vi "Keithley2450DrainS.vi"() -> ()   [LabVIEW 2025]
doc: "Author: Scott Hannahs <sth@magnet.fsu.edu>\n\nThis software is licensed for use under the “MIT License\"\nCopyright (c) 2025 Scott Hannahs, sth@sth@magnet.sthnet.net\n\nPermission is hereby granted, free of charge, to any person obtaining a copy of this software and associated documentation files (the \"Software\"), to deal in the Software without restriction, including without limitation the rights to use, copy, modify, merge, publish, distribute, sublicense, and/or sell copies of the Software, and to permit persons to whom the Software is furnished to do so, subject to the following conditions: The above copyright notice and this permission notice shall be included in all copies or substantial portions of the Software.\n\nTHE SOFTWARE IS PROVIDED \"AS IS\", WITHOUT WARRANTY OF ANY KIND, EXPRESS OR IMPLIED, INCLUDING BUT NOT LIMITED TO THE WARRANTIES OF MERCHANTABILITY, FITNESS FOR A PARTICULAR PURPOSE AND NONINFRINGEMENT. IN NO EVENT SHALL THE AUTHORS OR COPYRIGHT HOLDERS BE LIABLE FOR ANY CLAIM, DAMAGES OR OTHER LIABILITY, WHETHER IN AN ACTION OF CONTRACT, TORT OR OTHERWISE, ARISING FROM, OUT OF OR IN CONNECTION WITH THE SOFTWARE OR THE USE OR OTHER DEALINGS IN THE SOFTWARE."
panel:
  out "Sweep\nTime  (sec)":u32 format="%.1f"
  in  "Button:SetupBySoft":bool
  in  "Autozero:":bool
  out "Was paused":bool=TRUE
  in  "VISA resource name":refnum<visa-resource-name>="GPIB0::7::INSTR"
  in  "INFINITE RUN":bool
  in  "MODE:":enum32{"SAW /|/|/|", "TRINGLE /\\/\\/\\"}(radio)=enum."TRINGLE /\\/\\/\\"
  in  "Step |Volt| (abs.)":dbl=0.05 min=1e-06 max=0.1 format="%^.3e"
  in  "Delay (s)":dbl=1.0 min=0.1 max=100.0 format="%.3f"
  in  "Stop Volt":dbl=1.0 min=-10.0 max=10.0 format="%^.3e"
  in  "Start Sweep":bool
  out "Last index":i32
  in  "Compliance Current":dbl=0.1 format="%.3e"
  in  "Start Volt":dbl min=-10.0 max=10.0 format="%^.3e"
  in  "Setup":bool
  in  "Pause/Resume sweep":bool
  out "StartStorage":dbl min=-10.0 max=10.0 format="%^.3e"
  out "StopStorage":dbl=1.0 min=-10.0 max=10.0 format="%^.3e"
  in  "Button:Continue":bool
  in  "Button:SweepBySoft":bool
  out "Volt by Computer":dbl min=-10.0 max=10.0 format="%^.3e"
  in  "stop sweep":bool
  in  "Output Zero":bool
  # "Select name then start VI"
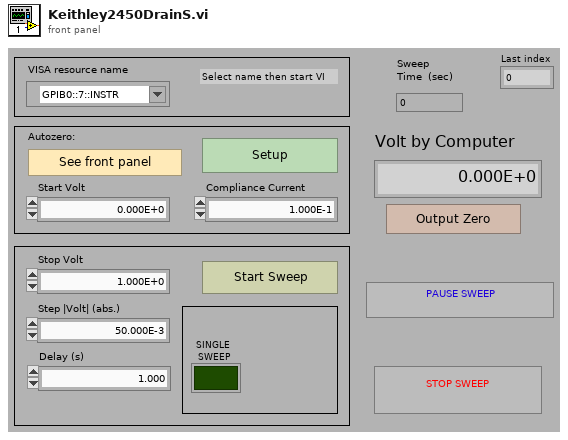
[diagram p1: front panel]
types:
  T1 = enum8{"Enabled", "Disabled", "Disabled and Grayed Out"}
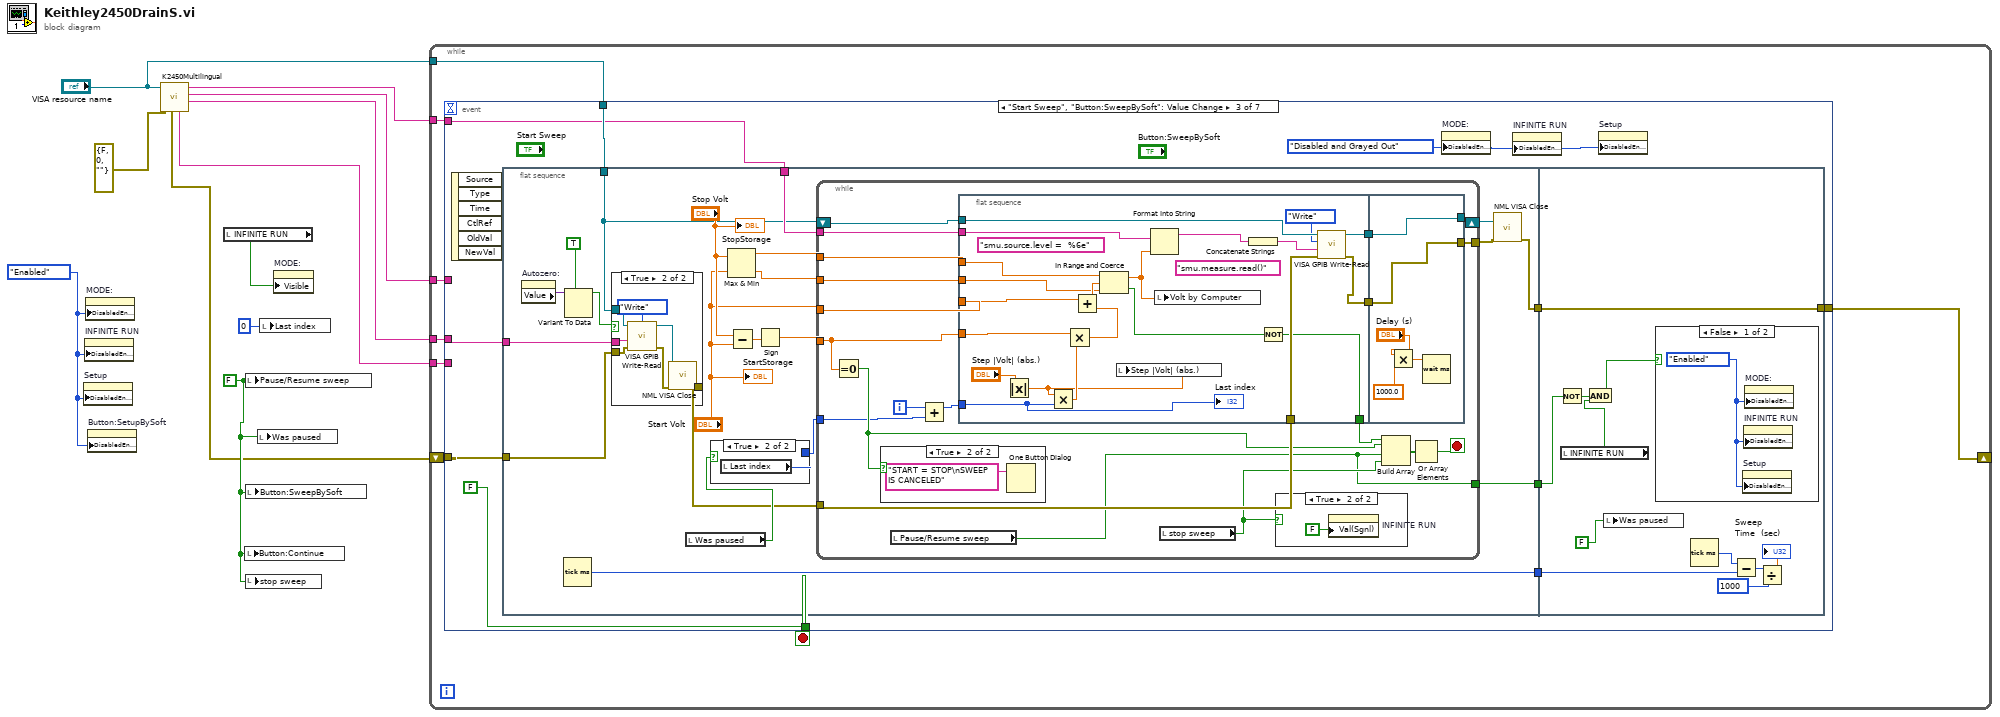
[diagram p0: block diagram]
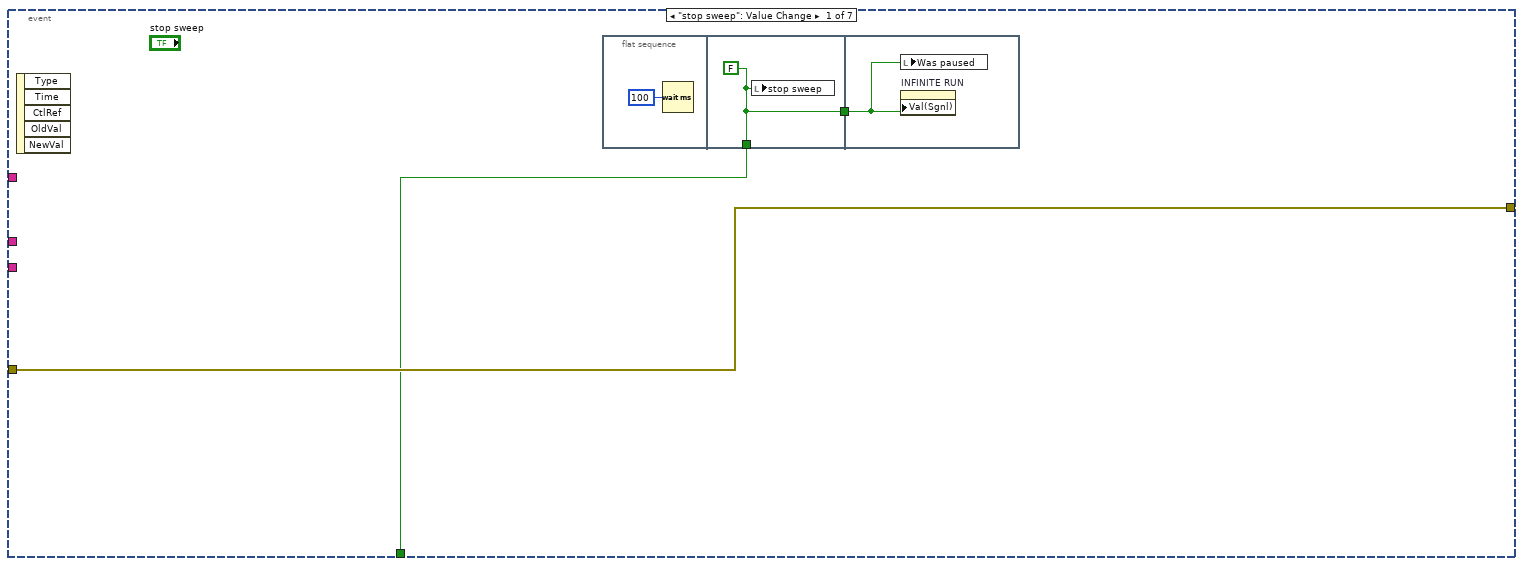
[diagram p2: hidden frame]
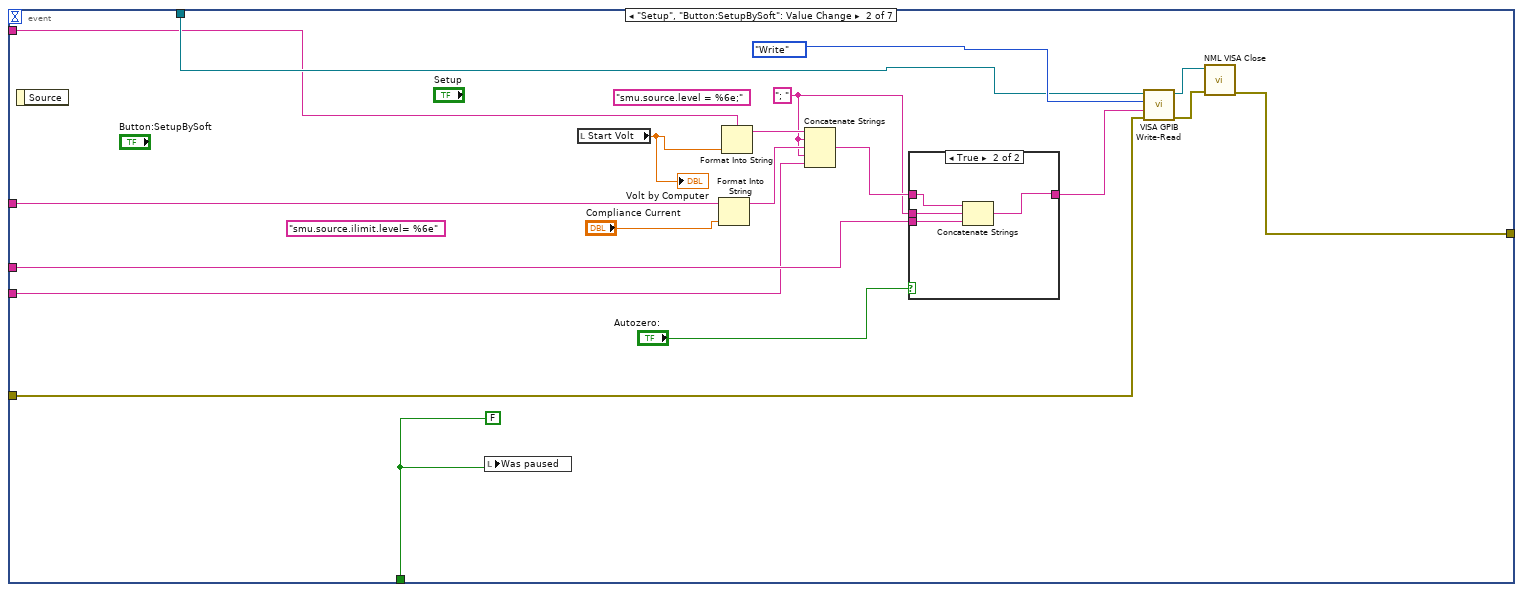
[diagram p3: hidden frame]
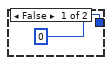
[diagram p6: hidden frame]
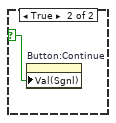
[diagram p9: hidden frame]
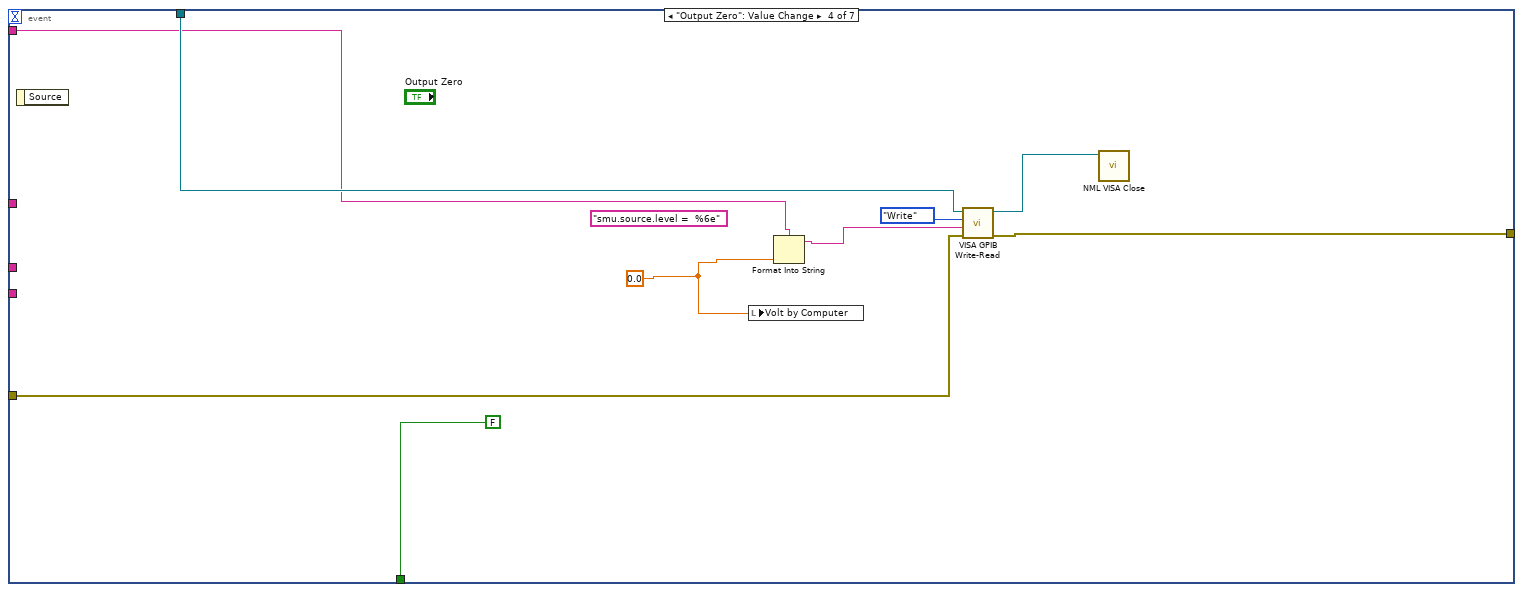
[diagram p10: hidden frame]
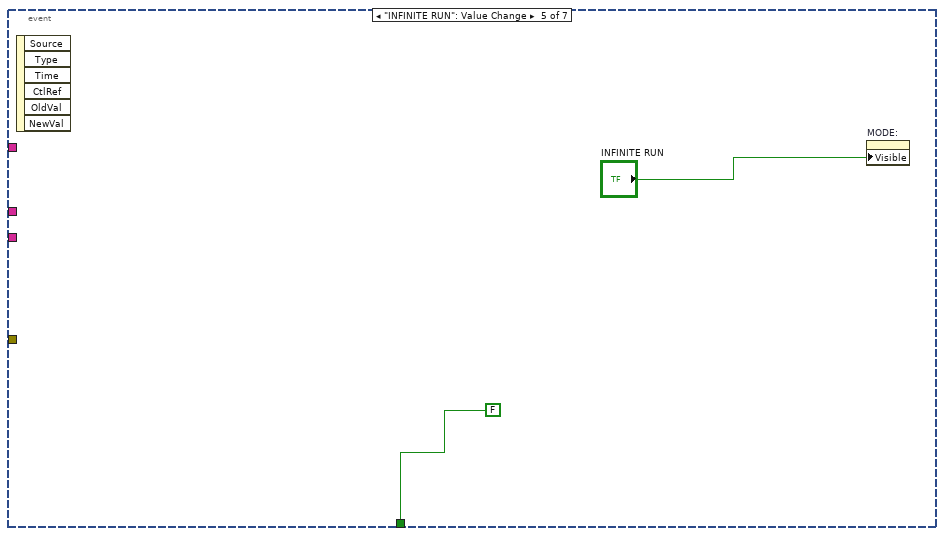
[diagram p11: hidden frame]
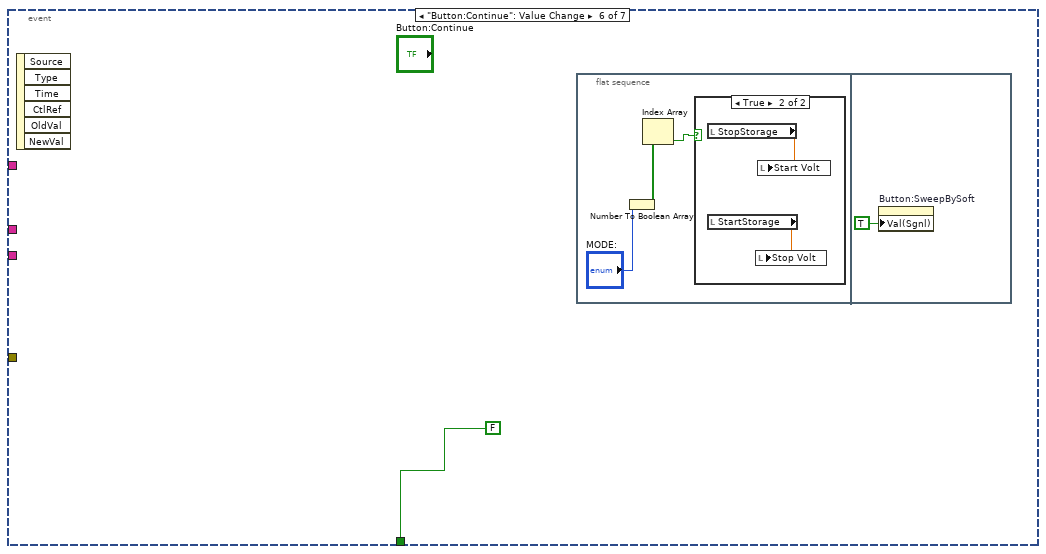
[diagram p12: hidden frame]
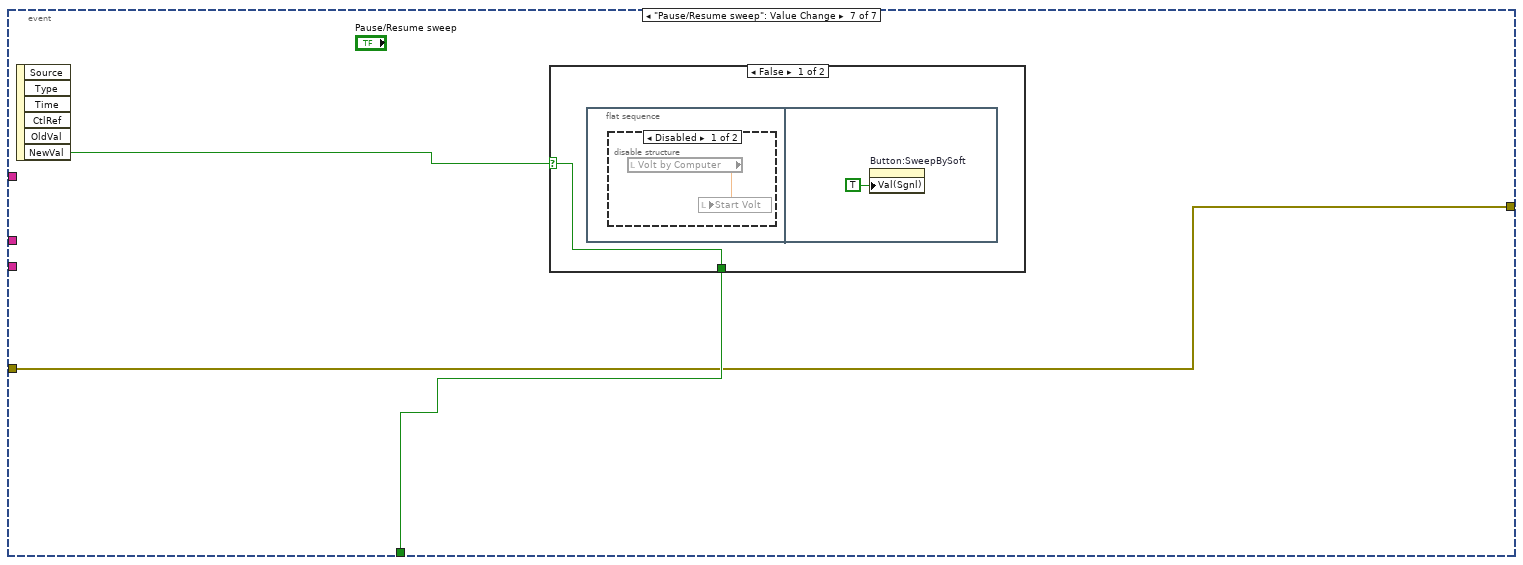
[diagram p14: hidden frame]
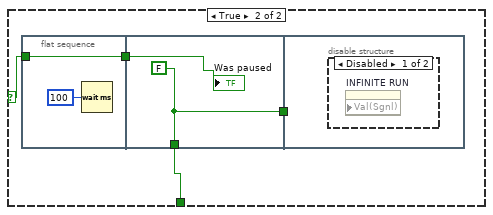
[diagram p16: hidden frame]
diagram:
  w2 = T1."Enabled" ("Disabled")
  w9 = FALSE ("Pause/Resume sweep")
  n1 = property on="Setup" class="Bool"("DisabledEnum"=w2) -> ()  [unwired: 2 in, 2 out]
  n2 = property on="INFINITE RUN" class="Bool (strict)"("DisabledEnum"=w2) -> ()  [unwired: 2 in, 2 out]
  n3 = property on="MODE:" class="RadioBtnsControl (strict)"("DisabledEnum"=w2) -> ()  [unwired: 2 in, 2 out]
  n4 = property on="Button:SetupBySoft" class="Bool (strict)"("DisabledEnum"=w2) -> ()  [unwired: 2 in, 2 out]
  n5 = call "K2450Multilingual.vi"("error in"=errorcluster {"status"=FALSE, "code"=0, "source"=""} ("error out"), "VISA resource name"="VISA resource name") -> ("AutozeroOnce"=w4:string, "Set Compliance"=w5:string, "Set Source Level"=w6:string, "Clear defbuffer1"=w1:string, "error out"=w7:errorcluster)  [unwired: 2 in, 2 out]
  n6 = local read "INFINITE RUN"() -> (w11:bool)
  n7 = local write "Button:Continue"(w9) -> ()
  n8 = local write "Pause/Resume sweep"(w9) -> ()
  n9 = local write "Button:SweepBySoft"(w9) -> ()
  n10 = local write "stop sweep"(w9) -> ()
  n11 = local write "Was paused"(w9) -> ()
  n12 = local write "Last index"(0 ("Last index")) -> ()
  n13 = property on="MODE:" class="RadioBtnsControl (strict)"("Visible"=w11) -> ()  [unwired: 2 in, 2 out]
  n14 = while {
    shift-right: [w18] -> _
    shift-left: w7 -> [w17]
    tunnel: "VISA resource name" -> [w16]
    tunnel: w6 -> [w15]
    tunnel: w5 -> [w14]
    tunnel: w4 -> [w13]
    tunnel: w1 -> [w12]
    stop <- w19 stop-if-true
    n15 = event shown="[2] \"Start Sweep\", \"Button:SweepBySoft\": Value Change" {
      selector: _ -> [_ _ _ _ _ _ _]
      dyn-events: _ -> [_ _ _ _ _ _ _]
      timeout: _ -> [_ _ _ _ _ _ _]
      tunnel: w16 -> [_ w38 w59 w159 _ _ _]
      tunnel: [w21 w35 FALSE ("NewVal") FALSE ("NewVal") FALSE ("NewVal") FALSE ("NewVal") w172] -> w19
      tunnel: [w22 w40 w57 w158 _ _ w171] -> w18
      tunnel: w17 -> [w22 w37 w58 w157 _ _ w171]
      tunnel: w15 -> [_ w33 w52 w152 _ _ _]
      tunnel: w14 -> [_ w32 _ _ _ _ _]
      tunnel: w13 -> [_ w28 w51 _ _ _ _]
      tunnel: w12 -> [_ w27 _ _ _ _ _]
      event "stop sweep": Value Change {
        n16 = event-data() -> ()  [unwired: 1 in, 5 out]
        n17 = flat-sequence {
          tunnel: [w24] -> w21
          tunnel: [w24] -> w20
          tunnel: w20 -> [w25]
          frame #0 {
            n18 = Wait (ms)(milliseconds to wait=u32 100) -> ()  [unwired: 1 out]
          }
          frame #1 {
            w24 = FALSE ("stop")
            n19 = local write "stop sweep"(w24) -> ()
          }
          frame #2 {
            n20 = local write "Was paused"(w25) -> ()
            n21 = property on="INFINITE RUN" class="Bool (strict)"("Val(Sgnl)"=w25) -> ()  [unwired: 2 in, 2 out]
          }
        }
      }
      event "Setup", "Button:SetupBySoft": Value Change {
        (unwired) "smu.source.ilimit.level= %6e"
        w26 = "; " ("string")
        w35 = FALSE ("NewVal")
        (unwired) "smu.source.level = %6e;"
        n22 = event-data() -> ()  [unwired: 1 in, 1 out]
        n23 = local write "Was paused"(w35) -> ()
        n24 = local read "Start Volt"() -> (w44:dbl)
        "Volt by Computer" <- w44
        n25 = Format Into String(format string=w32, "Compliance Current") -> (resulting string=w34:string)  [unwired: 2 in, 1 out]
        n26 = Format Into String(format string=w33, w44) -> (resulting string=w36:string)  [unwired: 2 in, 1 out]
        n27 = Concatenate Strings(w36, w26, w34, w26, w27) -> (w30:string)
        n28 = case shown="True" "Autozero:" {
          tunnel: w30 -> [w45 w49]
          tunnel: [w45 w46] -> w29
          tunnel: w26 -> [_ w48]
          tunnel: w28 -> [_ w47]
          frame False {
          }
          frame True {
            n29 = Concatenate Strings(w49, w48, w47) -> (w46:string)
          }
        }
        n30 = call "VISA GPIB Write-Read.vi"("error in (no error)"=w37, "Command"=w29, "Action"=enum16{"Write", "Read", "Write & Read"}."Write", "VISA resource name"=w38) -> ("error out"=w41:errorcluster, "dup VISA Session"=w42:refnum<visa-resource-name>)  [unwired: 4 in, 2 out]
        n31 = call "NML VISA Close.vi"("Error In"=w41, "VISA resource name"=w42) -> ("Error Out"=w40:errorcluster)  [unwired: 9 in]
      }
      event "Start Sweep", "Button:SweepBySoft": Value Change {
        w53 = T1."Disabled and Grayed Out" ("Disabled")
        n32 = event-data() -> ()  [unwired: 1 in, 6 out]
        n33 = flat-sequence {
          tunnel: w59 -> [w64]
          tunnel: [w74] -> w55
          tunnel: [w69] -> w54
          tunnel: w52 -> [w68]
          tunnel: w58 -> [w67]
          tunnel: w51 -> [w65]
          tunnel: [w60] -> w50
          tunnel: [w149] -> w57
          tunnel: w55 -> [w149]
          tunnel: w54 -> [w145]
          tunnel: w50 -> [w139]
          frame #0 {
            n34 = property on="Autozero:" class="Bool"() -> ("Value"=w63:variant)  [unwired: 2 in, 2 out]
            n35 = Tick Count (ms)() -> (millisecond timer value=w60:u32)
            n36 = Variant To Data(type=TRUE, Variant=w63) -> (data=w61:bool)  [unwired: 1 in, 1 out]
            n37 = case shown="True" w61 {
              tunnel: w67 -> [w81 w87]
              tunnel: [w81 w85] -> w66
              tunnel: w65 -> [_ w84]
              tunnel: w64 -> [_ w82]
              frame False {
              }
              frame True {
                n38 = call "VISA GPIB Write-Read.vi"("error in (no error)"=w87, "Command"=w84, "Action"=enum16{"Write", "Read", "Write & Read"}."Write", "VISA resource name"=w82) -> ("error out"=w86:errorcluster, "dup VISA Session"=w83:refnum<visa-resource-name>)  [unwired: 4 in, 2 out]
                n39 = call "NML VISA Close.vi"("Error In"=w86, "VISA resource name"=w83) -> ("Error Out"=w85:errorcluster)  [unwired: 9 in]
              }
            }
            n40 = local read "Was paused"() -> (w71:bool)
            n41 = case shown="True" w71 {
              tunnel: [0 w90] -> w70
              frame False {
              }
              frame True {
                n42 = local read "Last index"() -> (w90:i32)
              }
            }
            n43 = Max & Min(x="Stop Volt", y="Start Volt") -> (max(x,y)=w80:dbl, min(x,y)=w79:dbl)
            n44 = Subtract(x="Stop Volt", y="Start Volt") -> (x-y=w76:dbl)
            n45 = Sign(1:w76) -> (0:w75:dbl)
            n46 = while {
              tunnel: w66 -> [w110]
              tunnel: "Start Volt" -> [w109]
              tunnel: w80 -> [w104]
              tunnel: w79 -> [w103]
              tunnel: w75 -> [w97]
              tunnel: [w101] -> w73
              shift-right: [w100] -> w72
              shift-left: w64 -> [w99]
              tunnel: w70 -> [w94]
              tunnel: [w92] -> w69
              tunnel: w68 -> [w91]
              i -> [w107]
              stop <- w106 stop-if-true
              n47 = Equal To 0?(x=w97) -> (x = 0?=w96:bool)
              n48 = case shown="True" w96 {
                frame False {
                }
                frame True {
                  n49 = One Button Dialog(message="START = STOP\nSWEEP IS CANCELED") -> ()  [unwired: 1 in, 1 out]
                }
              }
              n50 = local read "Pause/Resume sweep"() -> (w92:bool)
              n51 = Add(x=w107, y=w94) -> (x+y=w98:i32)
              n52 = flat-sequence {
                tunnel: w99 -> [w133]
                tunnel: w110 -> [w132]
                tunnel: w109 -> [w130]
                tunnel: [w127] -> w105
                tunnel: [w131] -> w108
                tunnel: w98 -> [w114]
                tunnel: w104 -> [w121]
                tunnel: w103 -> [w120]
                tunnel: w97 -> [w117]
                tunnel: [w116] -> w102
                tunnel: w91 -> [w113]
                tunnel: w108 -> [w135]
                tunnel: w102 -> [w134]
                tunnel: [w135] -> w101
                tunnel: [w134] -> w100
                frame #0 {
                  (unwired) "smu.measure.read()" ("string")
                  (unwired) "smu.source.level =  %6e"
                  n53 = Absolute Value(x="Step |Volt| (abs.)") -> (abs(x)=w119:dbl)
                  n54 = Multiply(x=w119, y=w114) -> (x*y=w123:dbl)
                  n55 = Multiply(x=w117, y=w123) -> (x*y=w118:dbl)
                  n56 = Add(x=w130, y=w118) -> (x+y=w129:dbl)
                  n57 = In Range and Coerce(upper limit=w121, x=w129, lower limit=w120) -> (coerced(x)=w122:dbl, In Range?=w128:bool)
                  n58 = local write "Step |Volt| (abs.)"(w119) -> ()
                  n59 = Format Into String(format string=w113, w122) -> (resulting string=w126:string)  [unwired: 2 in, 1 out]
                  n60 = local write "Volt by Computer"(w122) -> ()
                  n61 = Concatenate Strings(w126) -> (w115:string)
                  n62 = Not(x=w128) -> (.not. x?=w127:bool)
                  n63 = call "VISA GPIB Write-Read.vi"("error in (no error)"=w132, "Command"=w115, "Action"=enum16{"Write", "Read", "Write & Read"}."Write", "VISA resource name"=w133) -> ("error out"=w131:errorcluster, "dup VISA Session"=w116:refnum<visa-resource-name>)  [unwired: 4 in, 2 out]
                  "Last index" <- w114
                }
                frame #1 {
                  n64 = Multiply(x="Delay (s)", y=1000.0) -> (x*y=w137:dbl)
                  n65 = Wait (ms)(milliseconds to wait=w137) -> ()  [unwired: 1 out]
                }
              }
              n66 = local read "stop sweep"() -> (w93:bool)
              n67 = case shown="True" w93 {
                frame False {
                }
                frame True {
                  n68 = property on="INFINITE RUN" class="Bool (strict)"("Val(Sgnl)"=FALSE ("Value (Signaling)")) -> ()  [unwired: 2 in, 2 out]
                }
              }
              n69 = Build Array(w105, w96, w92, w93) -> (w95:bool[])
              n70 = Or Array Elements(Boolean array=w95) -> (logical OR=w106:bool)
            }
            n71 = call "NML VISA Close.vi"("Error In"=w73, "VISA resource name"=w72) -> ("Error Out"=w74:errorcluster)  [unwired: 9 in]
            "StopStorage" <- "Stop Volt"
            "StartStorage" <- "Start Volt"
          }
          frame #1 {
            n72 = Not(x=w145) -> (.not. x?=w144:bool)
            n73 = local read "INFINITE RUN"() -> (w148:bool)
            n74 = And(x=w144, y=w148) -> (x .and. y?=w146:bool)
            n75 = local write "Was paused"(FALSE) -> ()
            n76 = case shown="False" w146 {
              selector: w146 -> [_ w151]
              frame False {
                w150 = T1."Enabled" ("Disabled")
                n77 = property on="Setup" class="Bool"("DisabledEnum"=w150) -> ()  [unwired: 2 in, 2 out]
                n78 = property on="INFINITE RUN" class="Bool (strict)"("DisabledEnum"=w150) -> ()  [unwired: 2 in, 2 out]
                n79 = property on="MODE:" class="RadioBtnsControl (strict)"("DisabledEnum"=w150) -> ()  [unwired: 2 in, 2 out]
              }
              frame True {
                n80 = property on="Button:Continue" class="Bool (strict)"("Val(Sgnl)"=w151) -> ()  [unwired: 2 in, 2 out]
              }
            }
            n81 = Tick Count (ms)() -> (millisecond timer value=w143:u32)
            n82 = Subtract(x=w143, y=w139) -> (x-y=w141:u32)
            n83 = Divide(x=w141, y=u32 1000) -> (x/y=→"Sweep\nTime  (sec)":dbl)
          }
        }
        n84 = property on="MODE:" class="RadioBtnsControl (strict)"("DisabledEnum"=w53) -> ()  [unwired: 2 in, 2 out]
        n85 = property on="INFINITE RUN" class="Bool (strict)"("DisabledEnum"=w53) -> ()  [unwired: 2 in, 2 out]
        n86 = property on="Setup" class="Bool"("DisabledEnum"=w53) -> ()  [unwired: 2 in, 2 out]
      }
      event "Output Zero": Value Change {
        w154 = 0.0 ("Output Volt 2")
        (unwired) "smu.source.level =  %6e"
        n87 = event-data() -> ()  [unwired: 1 in, 1 out]
        n88 = local write "Volt by Computer"(w154) -> ()
        n89 = Format Into String(format string=w152, w154) -> (resulting string=w155:string)  [unwired: 2 in, 1 out]
        n90 = call "VISA GPIB Write-Read.vi"("error in (no error)"=w157, "Command"=w155, "Action"=enum16{"Write", "Read", "Write & Read"}."Write", "VISA resource name"=w159) -> ("error out"=w158:errorcluster, "dup VISA Session"=w153:refnum<visa-resource-name>)  [unwired: 4 in, 2 out]
        n91 = call "NML VISA Close.vi"("VISA resource name"=w153) -> ()  [unwired: 10 in, 1 out]
      }
      event "INFINITE RUN": Value Change {
        n92 = event-data() -> ()  [unwired: 1 in, 6 out]
        n93 = property on="MODE:" class="RadioBtnsControl (strict)"("Visible"="INFINITE RUN") -> ()  [unwired: 2 in, 2 out]
      }
      event "Button:Continue": Value Change {
        n94 = event-data() -> ()  [unwired: 1 in, 6 out]
        n95 = flat-sequence {
          frame #0 {
            n96 = Number To Boolean Array(number="MODE:") -> (Boolean array=w166:bool[])
            n97 = Index Array(array=w166) -> (element=w164:bool)  [unwired: 1 in]
            n98 = case shown="True" w164 {
              frame False {
              }
              frame True {
                n99 = local read "StopStorage"() -> (w168:dbl)
                n100 = local read "StartStorage"() -> (w167:dbl)
                n101 = local write "Stop Volt"(w167) -> ()
                n102 = local write "Start Volt"(w168) -> ()
              }
            }
          }
          frame #1 {
            n103 = property on="Button:SweepBySoft" class="Bool (strict)"("Val(Sgnl)"=TRUE ("Value (Signaling)")) -> ()  [unwired: 2 in, 2 out]
          }
        }
      }
      event "Pause/Resume sweep": Value Change {
        n104 = event-data() -> ("NewVal"=w170:bool)  [unwired: 1 in, 5 out]
        n105 = case shown="False" w170 {
          selector: w170 -> [w173 w176]
          tunnel: [w173 w178] -> w172
          frame False {
            n106 = flat-sequence {
              frame #0 {
                n107 = disable-structure shown="Disabled" {
                  frame Disabled {
                    n108 = local read "Volt by Computer"() -> (w174:dbl)
                    n109 = local write "Start Volt"(w174) -> ()
                  }
                  frame Enabled {
                  }
                }
              }
              frame #1 {
                n110 = property on="Button:SweepBySoft" class="Bool (strict)"("Val(Sgnl)"=TRUE ("Value (Signaling)")) -> ()  [unwired: 2 in, 2 out]
              }
            }
          }
          frame True {
            n111 = flat-sequence {
              tunnel: [w180] -> w177
              tunnel: w176 -> [w180]
              tunnel: [w183] -> w178
              tunnel: [w183] -> w179
              tunnel: w177 -> [w182]
              tunnel: w179 -> [_]
              frame #0 {
                n112 = Wait (ms)(milliseconds to wait=u32 100) -> ()  [unwired: 1 out]
              }
              frame #1 {
                w183 = FALSE ("stop")
                "Was paused" <- w182
              }
              frame #2 {
                n113 = disable-structure shown="Disabled" {
                  frame Disabled {
                    n114 = property on="INFINITE RUN" class="Bool (strict)" props=["Val(Sgnl)"]() -> ()  [unwired: 3 in, 2 out]
                  }
                  frame Enabled {
                  }
                }
              }
            }
          }
        }
      }
    }
  }
